vi "countRate-sim.vi"() -> ()   [LabVIEW 2015]
doc: "This program is a simulation for radioactive decay countrate detection without an available DAQ. Gaussian noise generator is used to simulate a signal to demonstrate functionality."
uses:
  <vilib>/Platform/TimedLoop/XDataNode/timing_clust.ctl
  <vilib>/Platform/TimedLoop/XDataNode/nitl_modes.ctl
  <vilib>/Platform/TimedLoop/XDataNode/wakeup.ctl
  <vilib>/Utility/file.llb/Write Delimited Spreadsheet (I64).vi
  <vilib>/platform/TimedLoop/XDataNode/XDataNode.xnode
  <vilib>/Platform/TimedLoop/XDataNode/XDNodeRunTimeDep.lvlib
  <vilib>/Analysis/NI_AALBase.lvlib
panel:
  out "status":cluster{"Time Elapsed (sec)":i32, "Counts":dbl}={"Time Elapsed (sec)"=8, "Counts"=1.0} caption="COUNTING STATUS"
  in  "File Path Control":path=path "C:/Users/mylicon/Desktop/week8/sim-count-data"
  out "XY Graph":cluster{i32[], i32[]}(graph)={[0, 500, 1000, 1500, 2000, 2500, 3000, 3500, 4000, 4500, 5000, 5500, 6000, 6500, 7000, 7500, 8000, 8500, 9000, 9500, 10000, 10500, 11000, 11500, 12000, 12500, 13000, 13500, 14000, 14500, 15000, 15500, 16000, 16500, 17000, 17500, 18000, 18500, 19000, 19500, 20000, 20500, 21000, 21500, 22000, 22500, 23000, 23500, 24000, 24500, 25000, 25500, 26000, 26500, 27000, 27500, 28000, 28500, 29000, 29500, 30000], [1, 5, -4, 1, 0, -1, 3, -4, 0, 1, 2, 0, -2, -1, 0, 1, 1, -2, 1, 2, -3, 3, -3, 0, 2, -2, 0, 1, -1, 0, 3, -1, -1, -2, 2, 0, 1, 0, -2, 0, 1, 0, -1, 1, 1, -2, 0, 1, 1, -1, 2, -1, -2, 0, 1, -1, 6, -6, 3, -1, -2]}
  in  "USER CONTROLS":T1={"Total Time"=30, "Cnt Interval"=500, "SigGen Order"=2.0}
  in  "Stop Button":bool
  out "counts per interval":dbl(knob)=1.0 scale=0.0..100.0
  # "SIMULATION USES GAUSSIAN NOISE GENERATOR AS SOURCE"
  # "Demo count rate VI for Physics 434"
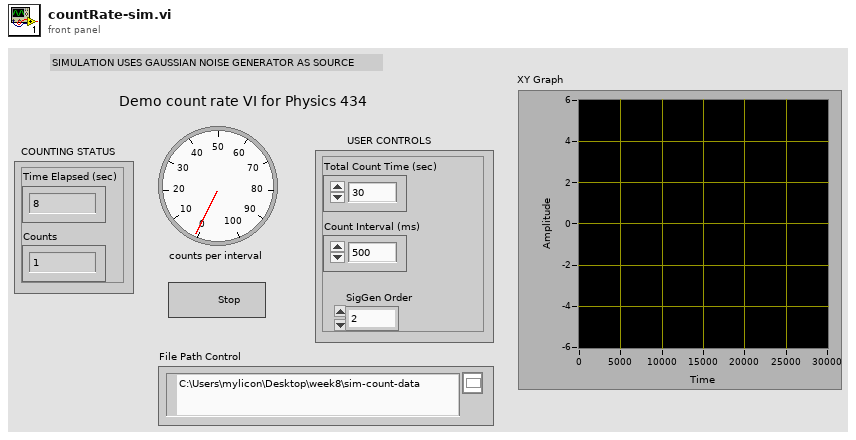
[diagram p1: front panel]
types:
  T1 = cluster{"Total Time":i32, "Cnt Interval":i32, "SigGen Order":dbl}
  T2 = typedef "XDNodeRunTimeDep.lvlib/timing_clust.ctl" = cluster{"Expected End [f-1]":u64, "Actual End [f-1]":u64, "Finished Late? [f-1]":bool, "Expected End [i-1]":u64, "Actual End [i-1]":u64, "Finished Late? [i-1]":bool, "Expected Start [i]":u64, "Actual Start [i]":u64, "Expected Start [f]":u64, "Actual Start [f]":u64, "Source Name":string, "Structure Name":string, "Period":i64, "Deadline":i64, "Offset":i64, "Start":i64, "Priority":i32, "Timeout":i32, "Mode":T3, "Wakeup Reason":T4, "Error":errorcluster, "Source Type":string, "Secondary Source Type":string, "Global End Time":u64, "Global Start Time":u64, "Frame Duration":u64, "Iteration Duration":u64, "Assigned CPU":i32, "I/O Scan Engine Mode":u32}
  T3 = typedef "XDNodeRunTimeDep.lvlib/nitl_modes.ctl" = enum32{"No Change", "Process missed periods, maintain original phase", "Discard missed periods, maintain original phase", "Process missed periods, ignore original phase", "Discard missed periods, ignore original phase"}
  T4 = typedef "XDNodeRunTimeDep.lvlib/wakeup.ctl" = enum32{"Normal", "Aborted", "Asynchronous wakeup", "Timing source error", "Timed loop error", "Timeout"}
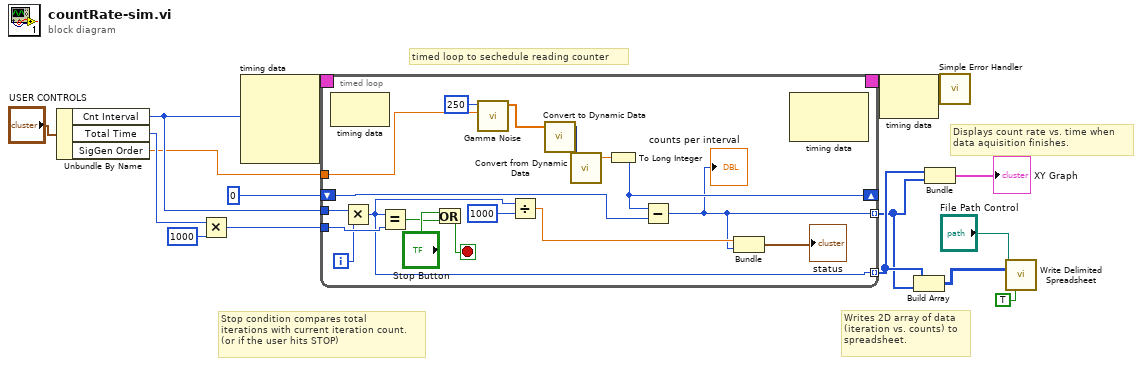
[diagram p0: block diagram]
diagram:
  # "Displays count rate vs. time when \ndata aquisition finishes."
  # "Writes 2D array of data \n(iteration vs. counts) to \nspreadsheet."
  # "Stop condition compares total \niterations with current iteration count. \n(or if the user hits STOP)"
  # "timed loop to sechedule reading counter"
  n1 = Unbundle By Name("USER CONTROLS") -> ("Cnt Interval"=w9:i32, "Total Time"=w11:i32, "SigGen Order"=w7:dbl)
  n2 = Multiply(x=w11, y=i64 1000) -> (x*y=w8:i64)
  n3 = node-c288(w9) -> (w16:T2)  [unwired: 3 in]
  n4 = timed-loop {
    timing: w16 -> [_]
    timing-out: [_] -> w15
    shift-right: [w33] -> _
    shift-left: 0 -> [w34]
    tunnel: w9 -> [w30]
    tunnel: w8 -> [w29]
    tunnel: w7 -> [w24]
    tunnel: [w17] -> w4 mode=indexing
    tunnel: [w20] -> w5 mode=indexing
    i -> [w22]
    stop <- w27 stop-if-true
    n5 = node-c288() -> ()  [unwired: 1 in, 1 out]
    n6 = Multiply(x=w30, y=w22) -> (x*y=w20:i32)
    n7 = Equal?(x=w20, y=w29) -> (x = y?=w28:bool)
    n8 = Or(x="Stop Button", y=w28) -> (x .or. y?=w27:bool)
    n9 = call <vilib>:"Gamma Noise.vi"("order"=w24, "samples"=250) -> ("gamma noise"=w26:dbl[])  [unwired: 8 in, 1 out]
    n10 = Divide(x=w20, y=1000) -> (x/y=w18:dbl)
    n11 = call "Convert to Dynamic Data"("Array"=w26) -> ("Dynamic Data Type"=w25:dynamicdata)  [unwired: 3 in]
    n12 = call "Convert from Dynamic Data"("Dynamic Data Type"=w25) -> ("Scalar"=w32:dbl)  [unwired: 3 in]
    n13 = To Long Integer(number=w32) -> (32bit integer=w33:i32)
    n14 = Subtract(x=w33, y=w34) -> (x-y=w17:i32)
    "counts per interval" <- w17
    n15 = Bundle(w18, w17) -> (→"status":cluster{dbl, i32})  [unwired: 1 in]
    n16 = node-c288() -> ()  [unwired: 2 in, 1 out]
  }
  n17 = node-c288(w15) -> (w13:errorcluster)
  n18 = Build Array(w5, w4) -> (w2:i32[][])
  n19 = Bundle(w5, w4) -> (→"XY Graph":cluster{i32[], i32[]})  [unwired: 1 in]
  n20 = call <vilib>:"Simple Error Handler.vi"("error in (no error)"=w13) -> ()  [unwired: 4 in, 5 out]
  n21 = call-poly <vilib>:"Write Delimited Spreadsheet.vi"("file path (dialog if empty)"="File Path Control", "2D data"=w2, "transpose? (F)"=TRUE) -> ()  [unwired: 11 in, 2 out]
